vi "recursive start.vi"() -> ()   [LabVIEW 2016]
panel:
  out "Sine":dynamicdata(graph)
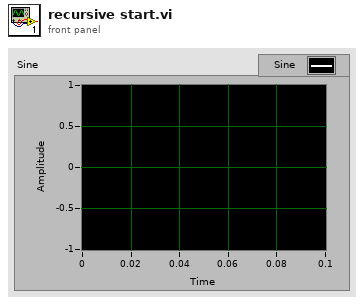
[diagram p1: front panel]
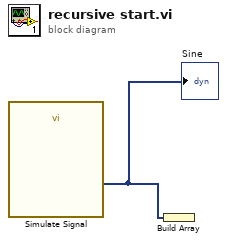
[diagram p0: block diagram]
diagram:
  n1 = call "Simulate Signal"() -> ("Sine"=w1:dynamicdata)  [unwired: 14 in, 1 out]
  "Sine" <- w1
  n2 = Build Array(w1) -> ()  [unwired: 1 out]
